vi "WPI_CameraRead MJPG for Dashboard.vi"(0 "Port":string="1181", 6 "Camera Settings":T5={"fps"=30, "compression"=30, "Image Size"=enum."320x240", "Config Shown"=FALSE}, 7 "Camera Settings 2":T3={"Exposure"=enum."Auto", "Exposure (%)"=50.0, "Brightness"=50, "White Balance"=enum."Auto", "Color Temp (K)"=0.0} {"Brightness" min=0 max=100}, 8 "Rec Mode":u16(ring) items=["O", "*", "Open Playback Panel"], 9 "Robot IP":string, 10 "Camera Name":string, 11 "Refnum in":T4) -> (2 "Active":bool, 3 "Refnum out":T4, 4 "FPS":dbl, 5 "Bandwidth (Mbps)":dbl)   [LabVIEW 2016]
doc: "This VI connects to a camera server at a given robot IP or device name. It requests images for a given camera name and settings. USB cameras should generally support all settings. IP cameras support only those in Camera Settings cluster. If the settings, name or other settings change, it will close and reopen as needed. The VI should be called repeatedly and it will fill in the image with the latest image from the server."
uses:
  <vilib>/Rock Robotics/WPI/Camera/WPI_CameraSettings Read MJPG.ctl
  <vilib>/Rock Robotics/WPI/Camera/WPI_CameraImageSize.ctl
  <vilib>/vision/Image Controls.llb/IMAQ Image.ctl
  <vilib>/Rock Robotics/WPI/Camera/WPI_CameraExposure Values.ctl
  <vilib>/Rock Robotics/WPI/Camera/WPI_CameraWhite Balance Values.ctl
  <vilib>/Rock Robotics/WPI/Dashboard/WPI_DashboardLogging Global.vi
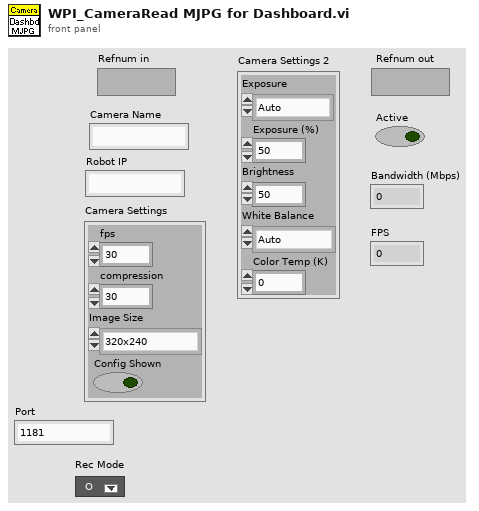
[diagram p1: front panel]
types:
  T1 = typedef "WPI_CameraExposure Values.ctl" = enum16{"Auto", "Flicker-free 50 Hz", "Flicker-free 60 Hz", "Hold current", "Custom"}
  T2 = typedef "WPI_CameraWhite Balance Values.ctl" = enum16{"Auto", "Fixed indoor", "Fixed outdoor 1", "Fixed outdoor 2", "Fixed fluorescent 1", "Fixed fluorescent 2", "Hold current", "Custom"}
  T3 = cluster{"Exposure":T1, "Exposure (%)":dbl, "Brightness":i32, "White Balance":T2, "Color Temp (K)":dbl}
  T4 = typedef "IMAQ Image.ctl" = refnum<image>
  T5 = typedef "WPI_CameraSettings Read MJPG.ctl" = cluster{"fps":i32, "compression":i32, "Image Size":T6, "Config Shown":bool}
  T6 = typedef "WPI_CameraImageSize.ctl" = enum16{"640x480", "320x240", "160x120", "Custom"}
  T7 = cluster{"token string":string, "token string 2":string}[]
  T8 = cluster{"Exposure":bool, "Exposure (%)":bool, "Brightness":bool, "White Balance":bool, "Color Temp (K)":bool}
  T9 = cluster{"token string":string, "token string":string}
  T10 = cluster{"token string":string, "token string":string}[]
  T11 = typedef "IMAQ AVI2 Refnum.ctl" = refnum<k20>
  T12 = cluster{"Camera Name":string, "fps":i32, "compression":i32, "Image Size":T6}
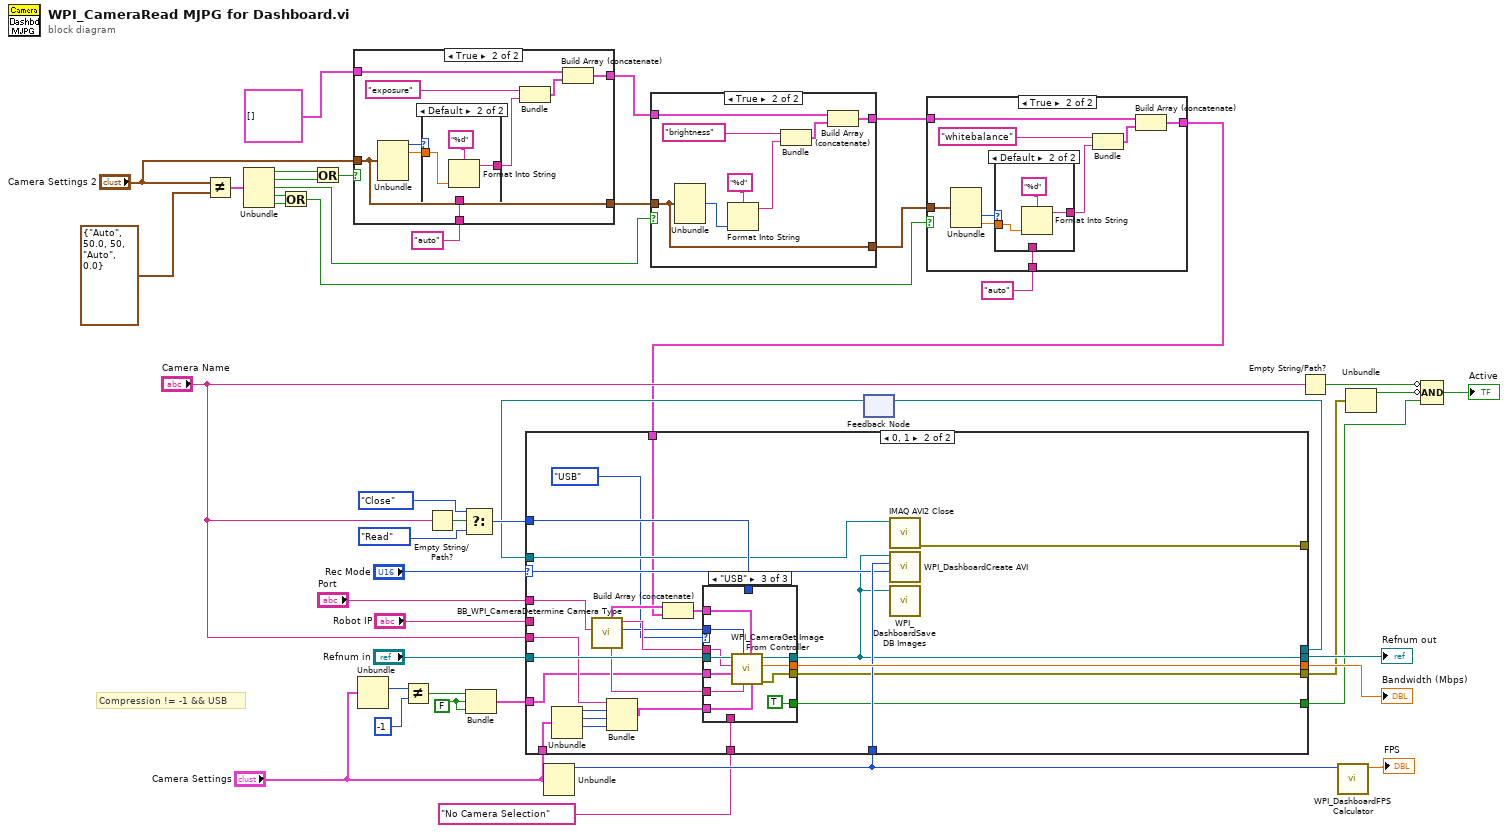
[diagram p0: block diagram]
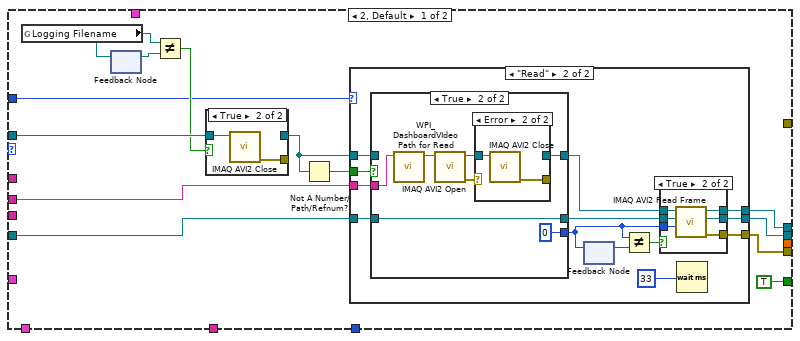
[diagram p7: hidden frame]
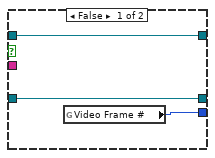
[diagram p10: hidden frame]
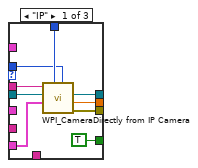
[diagram p13: hidden frame]
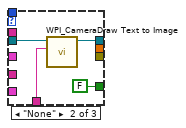
[diagram p14: hidden frame]
diagram:
  w22 = FALSE
  # "Compression != -1 && USB"
  n1 = Not Equal?(x="Camera Settings 2", y=T3 {"Exposure"=enum."Auto", "Exposure (%)"=50.0, "Brightness"=50, "White Balance"=enum."Auto", "Color Temp (K)"=0.0} ("Camera Settings 2")) -> (x != y?=w19:T8)
  n2 = Unbundle(w19) -> ("Exposure"=w17:bool, "Exposure (%)"=w16:bool, "Brightness"=w4:bool, "White Balance"=w8:bool, "Color Temp (K)"=w7:bool)
  n3 = Or(x=w8, y=w7) -> (x .or. y?=w6:bool)
  n4 = Or(x=w17, y=w16) -> (x .or. y?=w18:bool)
  n5 = case shown="True" w18 {
    tunnel: "Camera Settings 2" -> [w46 w48]
    tunnel: "auto" ("token string") -> [_ w53]
    tunnel: T7 [] ("parameters") -> [w47 w51]
    tunnel: [w47 w50] -> w13
    tunnel: [w46 w48] -> w10
    frame False {
    }
    frame True {
      n6 = Unbundle(w48) -> ("Exposure"=w55:T1, "Exposure (%)"=w54:dbl)  [unwired: 3 out]
      n7 = case shown="Default" w55 {
        tunnel: w54 -> [_ w60]
        tunnel: [w57 w59] -> w52
        tunnel: w53 -> [w57 _]
        frame "Auto" {
        }
        frame Default {
          n8 = Format Into String(format string="%d" ("token string"), w60) -> (resulting string=w59:string)  [unwired: 2 in, 1 out]
        }
      }
      n9 = Bundle("token string"="exposure", "token string"=w52) -> (w49:T9)  [unwired: 1 in]
      n10 = Build Array (concatenate)(w51, w49) -> (w50:T10)
    }
  }
  n11 = Unbundle("Camera Settings") -> ("compression"=w26:i32)  [unwired: 3 out]
  n12 = Not Equal?(x=w26, y=-1) -> (x != y?=w21:bool)
  n13 = Empty String/Path?(string/path="Camera Name") -> (empty?=w28:bool)
  n14 = Select(t=enum16{"Read", "Reopen", "Close"}."Close" ("Operation"), s=w28, f=enum16{"Read", "Reopen", "Close"}."Read" ("Operation")) -> (s? t:f=w42:enum16{"Read", "Reopen", "Close"})
  n15 = Bundle(w21, w22, w22) -> (w20:cluster{bool, bool, bool})  [unwired: 1 in]
  n16 = Unbundle("Camera Settings") -> ("fps"=w30:i32)  [unwired: 3 out]
  n17 = case shown="True" w4 {
    tunnel: w10 -> [w61 w64]
    tunnel: w13 -> [w62 w68]
    tunnel: [w62 w67] -> w11
    tunnel: [w61 w64] -> w9
    frame False {
    }
    frame True {
      n18 = Unbundle(w64) -> ("Brightness"=w63:i32)  [unwired: 4 out]
      n19 = Format Into String(format string="%d" ("token string"), w63) -> (resulting string=w69:string)  [unwired: 2 in, 1 out]
      n20 = Bundle("token string"="brightness", w69) -> (w66:cluster{"token string":string, string})  [unwired: 1 in]
      n21 = Build Array (concatenate)(w68, w66) -> (w67:T10)
    }
  }
  n22 = feedback #1() -> (w34:T11)  [unwired: 1 in]
  n23 = case shown="True" w6 {
    tunnel: w9 -> [_ w79]
    tunnel: "auto" ("token string") -> [_ w78]
    tunnel: w11 -> [w71 w76]
    tunnel: [w71 w75] -> w3
    frame False {
    }
    frame True {
      n24 = Unbundle(w79) -> ("White Balance"=w73:T2, "Color Temp (K)"=w72:dbl)  [unwired: 3 out]
      n25 = case shown="Default" w73 {
        tunnel: w72 -> [_ w84]
        tunnel: [w81 w83] -> w77
        tunnel: w78 -> [w81 _]
        frame "Auto" {
        }
        frame Default {
          n26 = Format Into String(format string="%d" ("token string"), w84) -> (resulting string=w83:string)  [unwired: 2 in, 1 out]
        }
      }
      n27 = Bundle("token string"="whitebalance", "token string"=w77) -> (w74:T9)  [unwired: 1 in]
      n28 = Build Array (concatenate)(w76, w74) -> (w75:T10)
    }
  }
  n29 = case shown="0, 1" "Rec Mode" {
    selector: "Rec Mode" -> [_ w158]
    tunnel: "Camera Settings" -> [_ w153]
    tunnel: w42 -> [w86 w162]
    tunnel: [_ w161] -> w39
    tunnel: [w97 w154] -> w35
    tunnel: "Refnum in" -> [w95 w160]
    tunnel: "Robot IP" -> [w92 _]
    tunnel: w30 -> [_ w159]
    tunnel: w34 -> [w90 w156]
    tunnel: [w94 _] -> w33
    tunnel: [w93 w157] -> w32
    tunnel: [_ w155] -> _
    tunnel: "Camera Name" -> [_ w146]
    tunnel: [TRUE w148] -> w24
    tunnel: "No Camera Selection" -> [_ w147]
    tunnel: w20 -> [_ w142]
    tunnel: w3 -> [_ w139]
    tunnel: "Port" -> [_ w137]
    frame 2, Default {
      n30 = global read "WPI_DashboardLogging Global.vi" "Logging Filename"() -> (w89:path)
      n31 = feedback #2() -> (w88:path)  [unwired: 1 in]
      n32 = feedback-in #2(w89) -> ()
      n33 = Not Equal?(x=w89, y=w88) -> (x != y?=w87:bool)
      n34 = case shown="True" w87 {
        tunnel: [w134 _] -> w91
        tunnel: w90 -> [w134 w136]
        tunnel: [_ w135] -> _
        frame False {
        }
        frame True {
          n35 = call "IMAQ AVI2 Close"("AVI Refnum"=w136) -> ("error out"=w135:errorcluster)  [unwired: 10 in]
        }
      }
      n36 = Not A Number/Path/Refnum?(number/path/refnum=w91) -> (NaN/Path/Refnum?=w96:bool)
      n37 = case shown="\"Read\"" w86 {
        tunnel: [w98 w112] -> w97
        tunnel: w96 -> [_ w111]
        tunnel: w95 -> [w98 w108]
        tunnel: [w99 w107] -> w94
        tunnel: [_ w106] -> w93
        tunnel: w92 -> [_ w105]
        tunnel: w91 -> [w99 w104]
        frame "Close", Default {
        }
        frame "Read" {
          n38 = case shown="True" w111 {
            tunnel: [w123 w128] -> w110
            tunnel: w104 -> [w123 _]
            tunnel: [w122 w130] -> w109
            tunnel: w108 -> [w122 w130]
            tunnel: [w121 0 ("Video Frame #")] -> w101
            tunnel: w105 -> [_ w125]
            frame False {
              n39 = global read "WPI_DashboardLogging Global.vi" "Video Frame #"() -> (w121:i32)
            }
            frame True {
              n40 = call <vilib>:"WPI_DashboardVIdeo Path for Read.vi"("Camera IP"=w125) -> ("Video Path"=w124:path)  [unwired: 10 in]
              n41 = call "IMAQ AVI2 Open"("AVI File Path"=w124) -> ("error out"=w129:errorcluster, "AVI Refnum"=w127:T11)  [unwired: 9 in]
              n42 = case shown="Error" w129 {
                tunnel: [w131 _] -> w128
                tunnel: w127 -> [w131 w133]
                tunnel: [_ w132] -> _
                frame No Error {
                }
                frame Error {
                  n43 = call "IMAQ AVI2 Close"("AVI Refnum"=w133) -> ("error out"=w132:errorcluster)  [unwired: 10 in]
                }
              }
            }
          }
          n44 = feedback #3() -> (w102:i32)  [unwired: 1 in]
          n45 = feedback-in #3(w101) -> ()
          n46 = Not Equal?(x=w101, y=w102) -> (x != y?=w103:bool)
          n47 = case shown="True" w103 {
            tunnel: [w113 w120] -> w112
            tunnel: w110 -> [w114 w119]
            tunnel: w109 -> [w113 w118]
            tunnel: [w114 w117] -> w107
            tunnel: [_ w116] -> w106
            tunnel: w101 -> [_ w115]
            frame False {
            }
            frame True {
              n48 = call "IMAQ AVI2 Read Frame"("Frame Number"=w115, "Image"=w118, "AVI Refnum"=w119) -> ("error out"=w116:errorcluster, "Image Out"=w120:T4, "AVI Refnum (duplicate)"=w117:T11)  [unwired: 6 in]
            }
          }
          n49 = Wait (ms)(milliseconds to wait=33) -> ()  [unwired: 1 out]
        }
      }
    }
    frame 0, 1 {
      n50 = Unbundle(w153) -> ("fps"=w150:i32, "compression"=w151:i32, "Image Size"=w152:T6)  [unwired: 1 out]
      n51 = call "BB_WPI_CameraDetermine Camera Type.vi"("Port"=w137) -> ("port"=w144:i32, "address"=w145:string, "cgi string"=w143:string, "parameters"=w140:T7)  [unwired: 7 in]
      n52 = Bundle("Camera Name"=w146, "fps"=w150, "compression"=w151, "Image Size"=w152) -> (w149:T12)  [unwired: 1 in]
      n53 = Build Array (concatenate)(w140, w139) -> (w141:T10)
      n54 = case shown="\"USB\"" enum16{"None", "USB", "IP"}."USB" ("Camera Type") {
        tunnel: w149 -> [w171 _ w182]
        tunnel: w162 -> [w165 _ _]
        tunnel: [w169 _ w181] -> w161
        tunnel: w160 -> [w167 w173 w186]
        tunnel: w145 -> [w166 _ w183]
        tunnel: [w170 _ w184] -> w157
        tunnel: [w168 w174 w185] -> w154
        tunnel: [TRUE FALSE TRUE] -> w148
        tunnel: w147 -> [_ w172 _]
        tunnel: w144 -> [w163 _ w179]
        tunnel: w143 -> [_ _ w177]
        tunnel: w142 -> [_ _ w178]
        tunnel: w141 -> [_ _ w176]
        frame "IP" {
          n55 = call <vilib>:"WPI_CameraDirectly from IP Camera.vi"("port"=w163, "Operation"=w165, "Camera Settings"=w171, "Image"=w167, "address"=w166) -> ("error out"=w170:errorcluster, "Bandwidth (Mbps)"=w169:dbl, "Image Out"=w168:T4)  [unwired: 4 in]
        }
        frame "None" {
          n56 = call <vilib>:"WPI_CameraDraw Text to Image.vi"("Text"=w172, "Refnum in"=w173) -> ("Refnum out"=w174:T4)  [unwired: 9 in]
        }
        frame "USB" {
          n57 = call <vilib>:"WPI_CameraGet Image From Controller.vi"("Camera Settings"=w182, "parameters"=w176, "cgi String"=w177, "port"=w179, "Options"=w178, "Controller Address"=w183, "Image"=w186) -> ("error out"=w184:errorcluster, "Bandwidth (Mbps)"=w181:dbl, "Image Out"=w185:T4)  [unwired: 2 in]
        }
      }
      n58 = call "IMAQ AVI2 Close"("AVI Refnum"=w156) -> ("error out"=w155:errorcluster)  [unwired: 10 in]
      n59 = call <vilib>:"WPI_DashboardCreate AVI.vi"("Recording"=w158, "frames per seconds"=w159, "Image"=w154) -> ()  [unwired: 9 in]
      n60 = call <vilib>:"WPI_DashboardSave DB Images.vi"("Image"=w154) -> ()  [unwired: 3 in]
    }
  }
  "Bandwidth (Mbps)" <- w39
  "Refnum out" <- w35
  n61 = feedback-in #1(w33) -> ()
  n62 = Empty String/Path?(string/path="Camera Name") -> (empty?=w31:bool)
  n63 = call <vilib>:"WPI_DashboardFPS Calculator.vi"("Average Count"=w30) -> ("fps"=→"FPS":dbl)  [unwired: 9 in, 1 out]
  n64 = Unbundle(w32) -> ("status"=w43:bool)  [unwired: 2 out]
  n65 = Compound Arithmetic op=AND(invert w31, invert w43, w24) -> (→"Active":bool)
